vi "Parse Asynch Telemetry.vi"(10 "Variant":variant) -> (2 "AsynchTLM":T1 {"Data" format="%04x"; "Length" format="%04x"; "Address" format="%04x"})   [LabVIEW 2019]
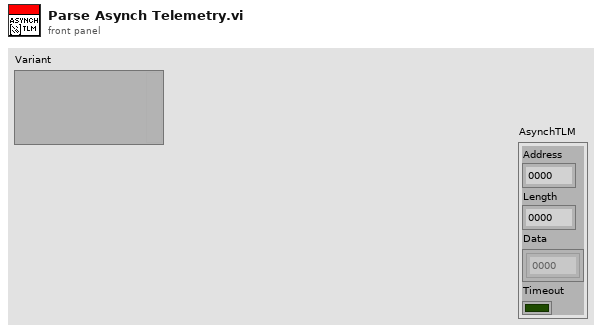
[diagram p1: front panel]
types:
  T1 = cluster{"Address":u16, "Length":u16, "Data":u16[], "Timeout":bool}
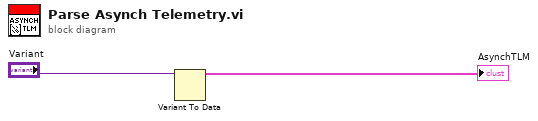
[diagram p0: block diagram]
diagram:
  n1 = Variant To Data(Variant="Variant") -> (data=→"AsynchTLM":T1)  [unwired: 2 in, 1 out]
